vi "RT_StepMotor_WP.vi"(9 "Direction":bool, 10 "Time between steps (ms)":i32=1, 11 "Steps":i64=1) -> ()   [LabVIEW 2014]
doc: "Random Laser Project\nAndré Romero - 2020\nandretec@ifsc.usp.br\n\nStep motor Control"
panel:
  # "DRV8825 Stepper Motor"
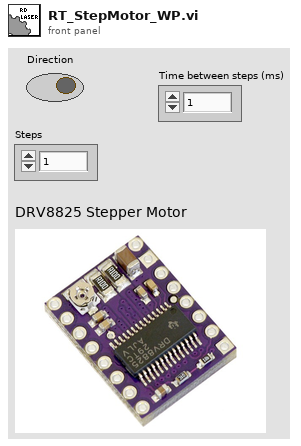
[diagram p1: front panel]
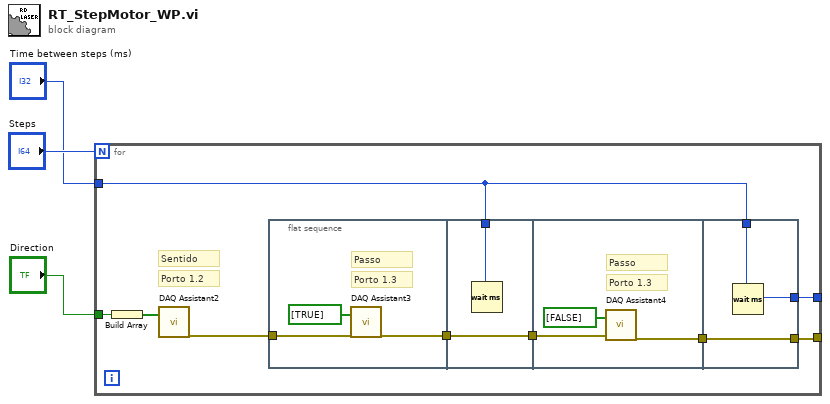
[diagram p0: block diagram]
diagram:
  n1 = for {
    N: "Steps" -> [_]
    tunnel: "Direction" -> [w11]
    tunnel: "Time between steps (ms)" -> [w9]
    tunnel: [w6] -> _
    tunnel: [w5] -> _
    # "Sentido"
    # "Porto 1.2"
    n2 = Build Array(w11) -> (w12:bool[])
    n3 = call "DAQ Assistant2"("data"=w12) -> ("error out"=w10:errorcluster)  [unwired: 17 in, 1 out]
    n4 = flat-sequence {
      tunnel: w10 -> [w15]
      tunnel: [w13] -> w8
      tunnel: w9 -> [w17]
      tunnel: w8 -> [w16]
      tunnel: [w16] -> w7
      tunnel: w7 -> [w19]
      tunnel: [w18] -> w4
      tunnel: w9 -> [w22]
      tunnel: [w22] -> w6
      tunnel: [w21] -> w5
      tunnel: w4 -> [w21]
      frame #0 {
        # "Passo"
        # "Porto 1.3"
        n5 = call "DAQ Assistant3"("data"=bool[] [TRUE], "error in"=w15) -> ("error out"=w13:errorcluster)  [unwired: 16 in, 1 out]
      }
      frame #1 {
        n6 = Wait (ms)(milliseconds to wait=w17) -> ()  [unwired: 1 out]
      }
      frame #2 {
        # "Passo"
        # "Porto 1.3"
        n7 = call "DAQ Assistant4"("data"=bool[] [FALSE], "error in"=w19) -> ("error out"=w18:errorcluster)  [unwired: 16 in, 1 out]
      }
      frame #3 {
        n8 = Wait (ms)(milliseconds to wait=w22) -> ()  [unwired: 1 out]
      }
    }
  }
